vi "Add Entry.vi"(5 "BG Color (None)":u32(colorbox), 7 "Name Prefix (none)":string, 8 "error in":errorcluster, 9 "Columns":string[](array[string]), 10 "Item":refnum<class "Item.lvclass">, 11 "Tree Map in":refnum<class "Project Tree Map.lvclass">) -> (0 "error out":errorcluster, 3 "Tree Map out":refnum<class "Project Tree Map.lvclass">)   [LabVIEW 2020, in "VI Properties Editor.lvlib" / "Project Tree Map.lvclass"]
doc: "Adds an entry to the tree map."
uses:
  Project Tree Map.lvclass
  Item/Item.lvclass
  Tree Entry.ctl
  <vilib>/picture/picture.llb/imagedata.ctl
  Project Tree Map.lvclass/Project Tree Map.ctl
  Tree Key.ctl
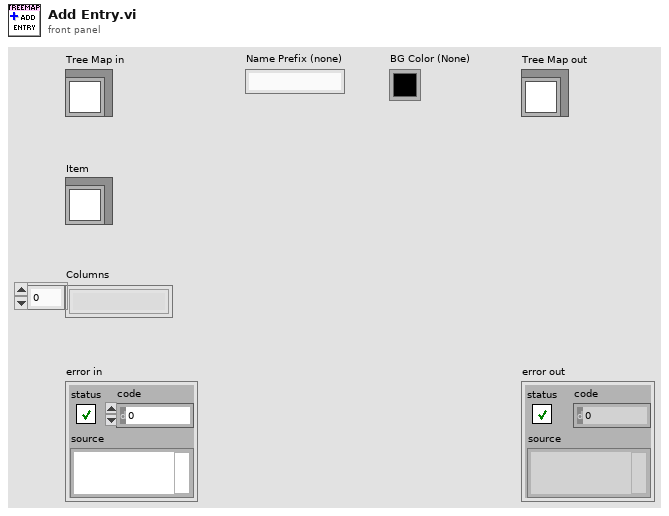
[diagram p1: front panel]
types:
  T1 = typedef "imagedata.ctl" = cluster{"image type":i32, "image depth":i32, "image":u8[], "mask":u8[], "colors":u32[], "Rectangle":cluster{"left":i16, "top":i16, "right":i16, "bottom":i16}}
  T2 = typedef "VI Properties Editor.lvlib/Project Tree Map.lvclass/Tree Entry.ctl" = cluster{"Hierarchy":string[], "Name":string, "Columns":string[], "BG Color":u32, "Leaf":bool, "Symbol":string, "Parent Tag":string, "Order":i32, "Tag":string}
  T3 = typedef "VI Properties Editor.lvlib/Project Tree Map.lvclass/Tree Key.ctl" = cluster{"Order":i32, "Hierarchy":string[]}
  T4 = map{string, cluster{"index":i32, "image data":T1}}
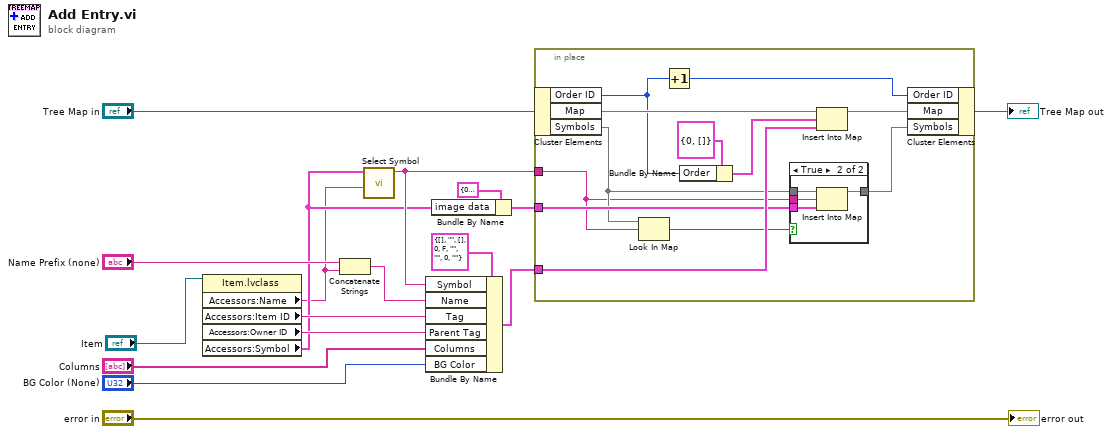
[diagram p0: block diagram]
diagram:
  n1 = property class="Item.lvclass"(reference="Item") -> ("Accessors:Name"=w1:string, "Accessors:Item ID"=w11:string, "Accessors:Owner ID"=w10:string, "Accessors:Symbol"=w3:T1)  [unwired: 1 in, 2 out]
  n2 = Concatenate Strings("Name Prefix (none)", w1) -> (w8:string)
  n3 = call "Select Symbol.vi"("Name"=w1, "Symbol"=w3) -> ("Symbol ID"=w6:string)  [unwired: 9 in]
  n4 = Bundle By Name(cluster=T2 {"Hierarchy"=[], "Name"="", "Columns"=[], "BG Color"=0, "Leaf"=FALSE, "Symbol"="", "Parent Tag"="", "Order"=0, "Tag"=""} ("Tree Entry"), "Symbol"=w6, "Name"=w8, "Tag"=w11, "Parent Tag"=w10, "Columns"="Columns", "BG Color"="BG Color (None)") -> (w5:T2)
  n5 = Bundle By Name(cluster=cluster{"index":i32, "image data":T1} {"index"=0, "image data"={"image type"=0, "image depth"=0, "image"=[], "mask"=[], "colors"=[], "Rectangle"={"left"=0, "top"=0, "right"=0, "bottom"=0}}} ("value"), "image data"=w3) -> (w2:cluster{"index":i32, "image data":T1})
  n6 = in-place {
    in-place-border: w6 -> [w19]
    in-place-border: w5 -> [w29]
    in-place-border: w2 -> [w21]
    n7 = in-place-cluster #1("Tree Map in") -> ("Order ID"=w24:i32, "Map"=w27:map{T3, T2}, "Symbols"=w20:T4)
    n8 = Look In Map(map=w20, key=w19) -> (key not found?=w18:bool)  [unwired: 1 in, 1 out]
    n9 = Increment(x=w24) -> (x+1=w23:i32)
    n10 = Bundle By Name(cluster=T3 {"Order"=0, "Hierarchy"=[]} ("key"), "Order"=w24) -> (w25:T3)
    n11 = case shown="True" w18 {
      tunnel: [w30 w34] -> w22
      tunnel: w21 -> [_ w33]
      tunnel: w20 -> [w30 w32]
      tunnel: w19 -> [_ w31]
      frame False {
      }
      frame True {
        n12 = Insert Into Map(map in=w32, key=w31, value=w33) -> (map out=w34:T4)  [unwired: 2 out]
      }
    }
    n13 = Insert Into Map(map in=w27, key=w25, value=w29) -> (map out=w28:map{T3, T2})  [unwired: 2 out]
    n14 = in-place-cluster #1("Order ID"=w23, "Map"=w28, "Symbols"=w22) -> (→"Tree Map out":refnum<class "Project Tree Map.lvclass">)
  }
  "error out" <- "error in"
